vi "SetAttributeViBoolean_SA-BP_CP_PS.vi"(7 "AttributeValue (Off)":bool, 8 "error in (no error)":errorcluster {"code" format="%.0x"}, 9 "AttributeID":u32(ring)=1150206 items=["SA_BURST_POWER_IF_GAIN_AUTO_ENABLED "=1150867, "SA_BURST_POWER_IF_GAIN_ENABLED "=1150866, "SA_BURSTPOWER_AVERAGE_ENABLED"=1150206, "SA_BURSTPOWER_BURST_WIDTH_AUTO_ENABLED"=1150194, "SA_BURSTPOWER_DISPLAY_BAR_GRAPH_ENABLED"=1150220, "SA_BURSTPOWER_DISPLAY_MAX_HOLD_ENABLED"=1150221, "SA_BURSTPOWER_DISPLAY_MIN_HOLD_ENABLED"=1150222, "SA_BURSTPOWER_DISPLAY_WINDOWX_AUTO_SCALE_ENABLED"=1150214, "SA_BURSTPOWER_DISPLAY_WINDOWY_AUTO_SCALE_ENABLED"=1150217, "SA_BURSTPOWER_MARKER_COUPLE_ENABLED"=1150244, "SA_BURSTPOWER_MARKER_ENABLED"=1150228, "SA_CHANNEL_POWER_POWER_LIMIT_ENABLED "=1150862, "SA_CHANNEL_POWER_PSD_LIMIT_ENABLED "=1150864, "SA_CHANNELPOWER_AVERAGE_ENABLED"=1150252, "SA_CHANNELPOWER_DETECTOR_TYPE_AUTO_ENABLED"=1150249, "SA_CHANNELPOWER_DISPLAY_BAR_GRAPH_ENABLED"=1150302, "SA_CHANNELPOWER_DISPLAY_WINDOWY_AUTO_SCALE_ENABLED"=1150301, "SA_CHANNELPOWER_FREQUENCY_PHASE_NOISE_OPTION_AUTO_ENABLED"=1150263, "SA_CHANNELPOWER_IF_GAIN_AUTO_ENABLED"=1150660, "SA_CHANNELPOWER_IF_GAIN"=1150659, "SA_CHANNELPOWER_MARKER_COUPLE_ENABLED"=1150279, "SA_CHANNELPOWER_MARKER_ENABLED"=1150282, "SA_CHANNELPOWER_OFFSETFILTER_ENABLED"=1150267, "SA_CHANNELPOWER_SWEEPCOUPLING_RESOLUTION_BANDWIDTH_AUTO_ENABLED"=1150258, "SA_CHANNELPOWER_SWEEPCOUPLING_SWEEP_TIME_AUTO_ENABLED"=1150273, "SA_CHANNELPOWER_SWEEPCOUPLING_VIDEO_BANDWIDTH_AUTO_ENABLED"=1150261, "SA_POWERSTATISTICS_DISPLAY_GAUSSIAN_LINE_ENABLED"=1150318, "SA_POWERSTATISTICS_DISPLAY_REFERENCE_TRACE_ENABLED"=1150338, "SA_POWERSTATISTICS_IF_GAIN_AUTO_ENABLED"=1150664, "SA_POWERSTATISTICS_IF_GAIN"=1150663, "SA_POWERSTATISTICS_MARKER_COUPLE_ENABLED"=1150348, "SA_POWERSTATISTICS_MARKER_ENABLED"=1150350], 11 "instrument handle":refnum<k15>) -> (0 "error out":errorcluster {"code" format="%.0x"}, 3 "instrument handle out":refnum<k15>)   [LabVIEW 2009, in "Keysight XSAn.lvlib"]
doc: "Sets a Boolean attribute from the instrument driver.\nThe following Attributes are supported:\n\nSA_BURST_POWER_IF_GAIN_AUTO_ENABLED \nSA_BURST_POWER_IF_GAIN_ENABLED \nSA_BURSTPOWER_AVERAGE_ENABLED\nSA_BURSTPOWER_BURST_WIDTH_AUTO_ENABLED\nSA_BURSTPOWER_DISPLAY_BAR_GRAPH_ENABLED\nSA_BURSTPOWER_DISPLAY_MAX_HOLD_ENABLED\nSA_BURSTPOWER_DISPLAY_MIN_HOLD_ENABLED\nSA_BURSTPOWER_DISPLAY_WINDOWX_AUTO_SCALE_ENABLED\nSA_BURSTPOWER_DISPLAY_WINDOWY_AUTO_SCALE_ENABLED\nSA_BURSTPOWER_MARKER_COUPLE_ENABLED\nSA_BURSTPOWER_MARKER_ENABLED\nSA_CHANNEL_POWER_POWER_LIMIT_ENABLED \nSA_CHANNEL_POWER_PSD_LIMIT_ENABLED \nSA_CHANNELPOWER_AVERAGE_ENABLED\nSA_CHANNELPOWER_DETECTOR_TYPE_AUTO_ENABLED\nSA_CHANNELPOWER_DISPLAY_BAR_GRAPH_ENABLED\nSA_CHANNELPOWER_DISPLAY_WINDOWY_AUTO_SCALE_ENABLED\nSA_CHANNELPOWER_FREQUENCY_PHASE_NOISE_OPTION_AUTO_ENABLED\nSA_CHANNELPOWER_IF_GAIN_AUTO_ENABLED\nSA_CHANNELPOWER_IF_GAIN\nSA_CHANNELPOWER_MARKER_COUPLE_ENABLED\nSA_CHANNELPOWER_MARKER_ENABLED\nSA_CHANNELPOWER_OFFSETFILTER_ENABLED\nSA_CHANNELPOWER_SWEEPCOUPLING_RESOLUTION_BANDWIDTH_AUTO_ENABLED\nSA_CHANNELPOWER_SWEEPCOUPLING_SWEEP_TIME_AUTO_ENABLED\nSA_CHANNELPOWER_SWEEPCOUPLING_VIDEO_BANDWIDTH_AUTO_ENABLED\nSA_POWERSTATISTICS_DISPLAY_GAUSSIAN_LINE_ENABLED\nSA_POWERSTATISTICS_DISPLAY_REFERENCE_TRACE_ENABLED\nSA_POWERSTATISTICS_IF_GAIN_AUTO_ENABLED\nSA_POWERSTATISTICS_IF_GAIN\nSA_POWERSTATISTICS_MARKER_COUPLE_ENABLED\nSA_POWERSTATISTICS_MARKER_ENABLED"
uses:
  <instrlib>/Keysight XSAn/Keysight XSAn.lvlib
  AgXSAn.dll
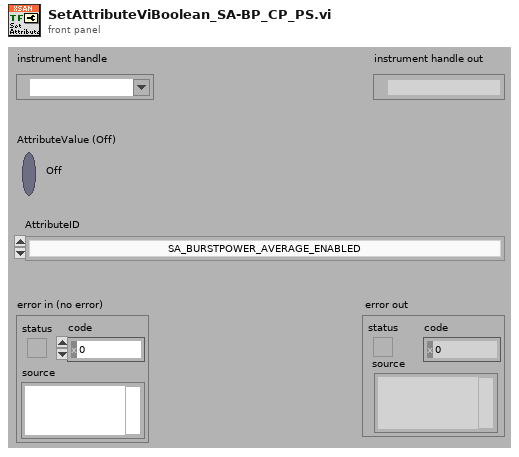
[diagram p1: front panel]
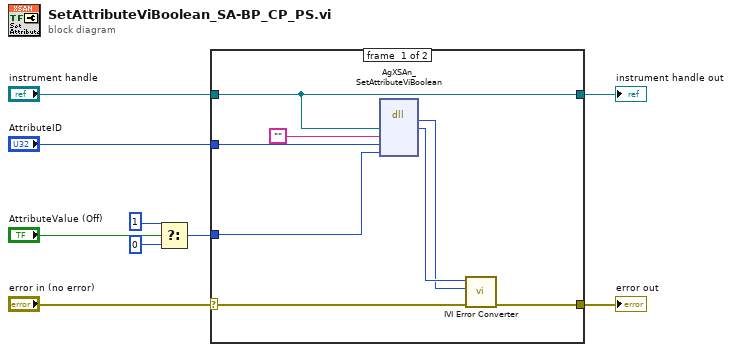
[diagram p0: block diagram]
diagram:
  n1 = Select(t=u16 1, s="AttributeValue (Off)", f=u16 0) -> (s? t:f=w2:u16)
  n2 = case shown="No Error" "error in (no error)" {
    selector: "error in (no error)" -> [w15 w19]
    tunnel: [w14 w19] -> w9
    tunnel: "instrument handle" -> [w11 w18]
    tunnel: "AttributeID" -> [w13 _]
    tunnel: w2 -> [w12 _]
    tunnel: [w11 w18] -> w1
    frame #0 {
      n3 = dll-call lib="AgXSAn**.dll" fn="AgXSAn_SetAttributeViBoolean"("Vi"=w11, "RepCapIdentifier"="", "AttributeID"=w13, "AttributeValue"=w12) -> ("return type"=w16:i32, "Vi"=w17:u32)  [unwired: 6 in, 2 out]
      n4 = call <instrlib>:"IVI Error Converter.vi"("error in (no error)"=w15, "IVI error code (0)"=w16, "instrument handle"=w17) -> ("error out"=w14:errorcluster)  [unwired: 7 in, 1 out]
    }
    frame #1 {
    }
  }
  "error out" <- w9
  "instrument handle out" <- w1
